vi "ParameterA Zone Checking.vi"(8 "error in (no error)":errorcluster, 9 "Impedance Z (10m)":dbl=0.01 min=0.01 max=100000000.0 format="%^.2e", 10 "Frequency (20)":dbl=20.0 min=20.0 max=1000000.0 format="%.2f", 11 "VISA resource name":refnum<visa-resource-name>) -> (0 "error out":errorcluster, 1 "Zone":i8, 3 "VISA resource name out":refnum<visa-resource-name>)   [LabVIEW 2015, in "Agilent 428X Series.lvlib"]
doc: "This VI is to find out the corresponding Parameter A value of Zone being used. User can verify the result from figure 9-4 on page 9-12. \n\nDisclaimer: All accuracy calculation VI's are not part of the original \n driver. They are provided for supplementry purpose only.\n If user desires very high accuracy data, please do or \n check the calculation seperately."
uses:
  Agilent 428X Series.lvlib
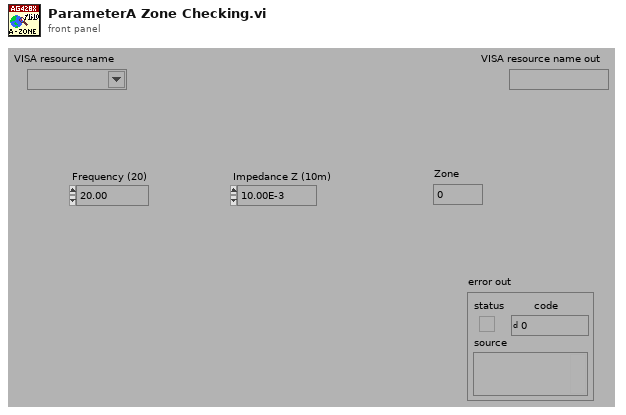
[diagram p1: front panel]
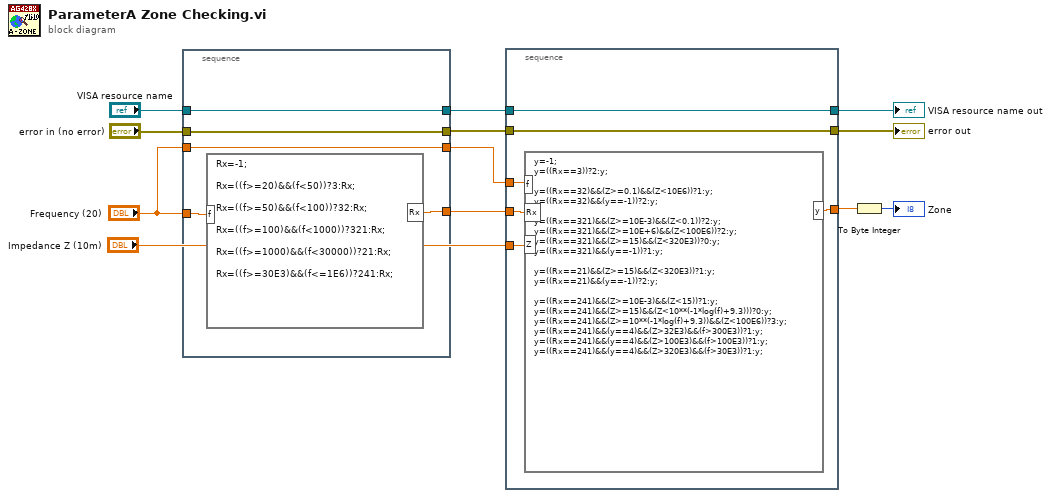
[diagram p0: block diagram]
diagram:
  n1 = stacked-sequence {
    tunnel: "VISA resource name" -> [w17]
    tunnel: [w17] -> w10
    tunnel: [w16] -> w9
    tunnel: "error in (no error)" -> [w16]
    tunnel: "Frequency (20)" -> [w15]
    tunnel: [w14] -> w5
    tunnel: "Frequency (20)" -> [w13]
    tunnel: [w13] -> w3
    frame #0 {
      n2 = formula code="Rx=-1;\n\nRx=((f>=20)&&(f<50))?3:Rx;\n\nRx=((f>=50)&&(f<100))?32:Rx;\n\nRx=((f>=100)&&(f<1000))?321:Rx;\n\nRx=((f>=1000)&&(f<30000))?21:Rx;\n\nRx=((f>=30E3)&&(f<=1E6))?241:Rx;"("f"=w15) -> ("Rx"=w14:dbl)
    }
  }
  n3 = stacked-sequence {
    tunnel: w10 -> [w22]
    tunnel: w9 -> [w23]
    tunnel: [w23] -> w8
    tunnel: [w22] -> w7
    tunnel: "Impedance Z (10m)" -> [w20]
    tunnel: w5 -> [w21]
    tunnel: [w19] -> w2
    tunnel: w3 -> [w18]
    frame #0 {
      n4 = formula code="y=-1;\ny=((Rx==3))?2:y;\n\ny=((Rx==32)&&(Z>=0.1)&&(Z<10E6))?1:y;\ny=((Rx==32)&&(y==-1))?2:y;\n\ny=((Rx==321)&&(Z>=10E-3)&&(Z<0.1))?2:y;\ny=((Rx==321)&&(Z>=10E+6)&&(Z<100E6))?2:y;\ny=((Rx==321)&&(Z>=15)&&(Z<320E3))?0:y;\ny=((Rx==321)&&(y==-1))?1:y;\n\ny=((Rx==21)&&(Z>=15)&&(Z<320E3))?1:y;\ny=((Rx==21)&&(y==-1))?2:y;\n\ny=((Rx==241)&&(Z>=10E-3)&&(Z<15))?1:y;\ny=((Rx==241)&&(Z>=15)&&(Z<10**(-1*log(f)+9.3)))?0:y;\ny=((Rx==241)&&(Z>=10**(-1*log(f)+9.3))&&(Z<100E6))?3:y;\ny=((Rx==241)&&(y==4)&&(Z>32E3)&&(f>300E3))?1:y;\ny=((Rx==241)&&(y==4)&&(Z>100E3)&&(f>100E3))?1:y; y=((Rx==241)&&(y==4)&&(Z>320E3)&&(f>30E3))?1:y;"("Rx"=w21, "Z"=w20, "f"=w18) -> ("y"=w19:dbl)
    }
  }
  "error out" <- w8
  "VISA resource name out" <- w7
  n5 = To Byte Integer(number=w2) -> (8bit integer=→"Zone":i8)
